vi "Min-Max.vi"() -> ()   [LabVIEW 2015]
uses:
  <vilib>/Utility/file.llb/Read Delimited Spreadsheet (DBL).vi
panel:
  out "Min Deðer":dbl
  out "Veriler":dbl[][](array[numeric])
  in  "Okunacak Veri Adresi":path
  out "Max Deðer":dbl
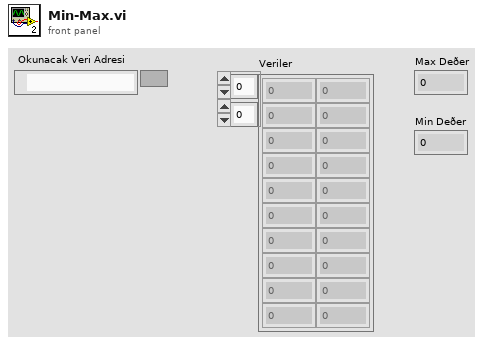
[diagram p1: front panel]
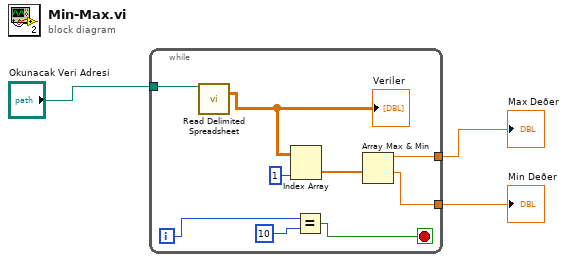
[diagram p0: block diagram]
diagram:
  n1 = while {
    tunnel: "Okunacak Veri Adresi" -> [w12]
    tunnel: [w5] -> w2
    tunnel: [w4] -> w1
    i -> [w10]
    stop <- w8 stop-if-true
    n2 = call-poly <vilib>:"Read Delimited Spreadsheet.vi"("file path (dialog if empty)"=w12) -> ("all rows"=w11:dbl[][])  [unwired: 9 in, 5 out]
    "Veriler" <- w11
    n3 = Index Array(array=w11, index (col)=1 ("disabled index (col)")) -> (element=w6:dbl[])  [unwired: 1 in]
    n4 = Equal?(x=w10, y=10) -> (x = y?=w8:bool)
    n5 = Array Max & Min(array=w6) -> (max value=w5:dbl, min value=w4:dbl)  [unwired: 2 out]
  }
  "Max Deðer" <- w2
  "Min Deðer" <- w1
